vi "PhaseNoise.vi"() -> ()   [LabVIEW 2009]
uses:
  <vilib>/imath/engines/lvmath2/RunTimeEngine/ErrorHandling/NIMS_Finalize Error.vi
  <vilib>/imath/engines/lvmath2/RunTimeEngine/Parser/MC_Version.vi
  <vilib>/imath/engines/lvmath2/RunTimeEngine/NodeEndStatement/NIMS_NodeEndStatement_Output.vi
  <instcachedir>/0/NIMS_NodeEndStatement_Output_53EC0D466D134D7ABD903AC30B43404B.lvgen/NIMS_NodeEndStatement_Output_53EC0D466D134D7ABD903AC30B43404B_001.vi
  <instcachedir>/0/NIMS_NodeEndStatement_Output_53EC0D466D134D7ABD903AC30B43404B.lvgen/NIMS_NodeEndStatement_Output_53EC0D466D134D7ABD903AC30B43404B_000.vi
  <vilib>/imath/engines/lvmath/Functions/Error Handling/MergeErrorsWrapper.vi
  <vilib>/imath/engines/lvmath2/RunTimeEngine/NodeEndStatement/NIMS_NodeEndStatement_Get Vector.vi
  <instcachedir>/0/NIMS_NodeEndStatement_Get Vector_708AE642CFEE4B9892E482CBBBA3A4D6.lvgen/NIMS_NodeEndStatement_Get Vector_708AE642CFEE4B9892E482CBBBA3A4D6_001.vi
  <vilib>/imath/engines/lvmath/Plug In/_Char/NIMS_CH_character datatype.ctl
  <vilib>/imathl/engines/lvmath/Functions/Error Handling/Create Error.vi
  <vilib>/imath/engines/lvmath2/RunTimeEngine/BuiltInFunctions/random/NIMS_random.vi
  <vilib>/imath/engines/lvmath/Plug In/_Char/NIMS_CH_Character RV to String.vi
  <vilib>/imath/engines/lvmath2/RunTimeEngine/RangeToken/NIMS_Range.vi
  <instcachedir>/0/NIMS_Range_08574DECC23E450FAF0AC0BC39E6BEA7.lvgen/NIMS_Range_08574DECC23E450FAF0AC0BC39E6BEA7_001.vi
  <vilib>/imath/engines/lvmath/Functions/Error Handling/MC_Error Cluster From Error Code.vi
  <vilib>/imath/engines/lvmath2/RunTimeEngine/BuiltInFunctions/fft/NIMS_fft(GV).vi
  <instcachedir>/0/NIMS_fft(GV)_4C6467FC22F84E4BA42517A07EF978B0.lvgen/NIMS_fft(GV)_4C6467FC22F84E4BA42517A07EF978B0_001.vi
  <vilib>/imath/engines/lvmath2/RunTimeEngine/BuiltInFunctions/abs/NIMS_abs(signed).vi
  <instcachedir>/0/NIMS_abs(signed)_C4FCB8E6058B49B797C7C8D53CA5F6EC.lvgen/NIMS_abs(signed)_C4FCB8E6058B49B797C7C8D53CA5F6EC_000.vi
  <vilib>/imath/engines/lvmath2/RunTimeEngine/VariableToken/Read/NIMS_Get Elements - RV(_) - Check(_).vi
  <instcachedir>/0/NIMS_Get Elements - RV(_) - Check(_)_FD08F12CA9A340B3A4DC1D5FF02404A0.lvgen/NIMS_Get Elements - RV(_) - Check(_)_FD08F12CA9A340B3A4DC1D5FF02404A0_001.vi
  <vilib>/imath/engines/lvmath2/RunTimeEngine/VariableToken/Read/NIMS_Get Elements - RV(_) - Check.vi
  <instcachedir>/0/NIMS_Get Elements - RV(_) - Check_30A5434E2C4242B098C990FE3FB371BC.lvgen/NIMS_Get Elements - RV(_) - Check_30A5434E2C4242B098C990FE3FB371BC_001.vi
  <instcachedir>/0/NIMS_Get Elements - RV(_) - Check(_)_FD08F12CA9A340B3A4DC1D5FF02404A0.lvgen/NIMS_Get Elements - RV(_) - Check(_)_FD08F12CA9A340B3A4DC1D5FF02404A0_002.vi
  <instcachedir>/0/NIMS_Get Elements - RV(_) - Check_30A5434E2C4242B098C990FE3FB371BC.lvgen/NIMS_Get Elements - RV(_) - Check_30A5434E2C4242B098C990FE3FB371BC_002.vi
  <vilib>/imath/engines/lvmath2/RunTimeEngine/ArithmeticOperatorToken/NIMS_ArithmeticOperator_plus.vi
  <instcachedir>/0/NIMS_ArithmeticOperator_plus_48B9519178ED42D7840F01273E784BFE.lvgen/NIMS_ArithmeticOperator_plus_48B9519178ED42D7840F01273E784BFE_008.vi
  <vilib>/imath/engines/lvmath2/RunTimeEngine/BuiltInFunctions/fft/NIMS_fft(GM).vi
  <instcachedir>/0/NIMS_fft(GM)_D61006EB97DF48D4B7BC0A22887DF931.lvgen/NIMS_fft(GM)_D61006EB97DF48D4B7BC0A22887DF931_000.vi
  <instcachedir>/0/NIMS_abs(signed)_C4FCB8E6058B49B797C7C8D53CA5F6EC.lvgen/NIMS_abs(signed)_C4FCB8E6058B49B797C7C8D53CA5F6EC_002.vi
panel:
  out "Total Power (Watt)":dbl
  out "Power Imbalance (dB)":dbl
  out "Total Power (dB)":dbl
  out "Voltage Imbalance (dB)":dbl
  out "Signal + Noise Power (dB)":dbl[](graph)
  out "Signal Power (Watts)":dbl[](graph)
  out "Signal (Time Domain)":dbl[](graph)
  in  "N1":dbl=64.0
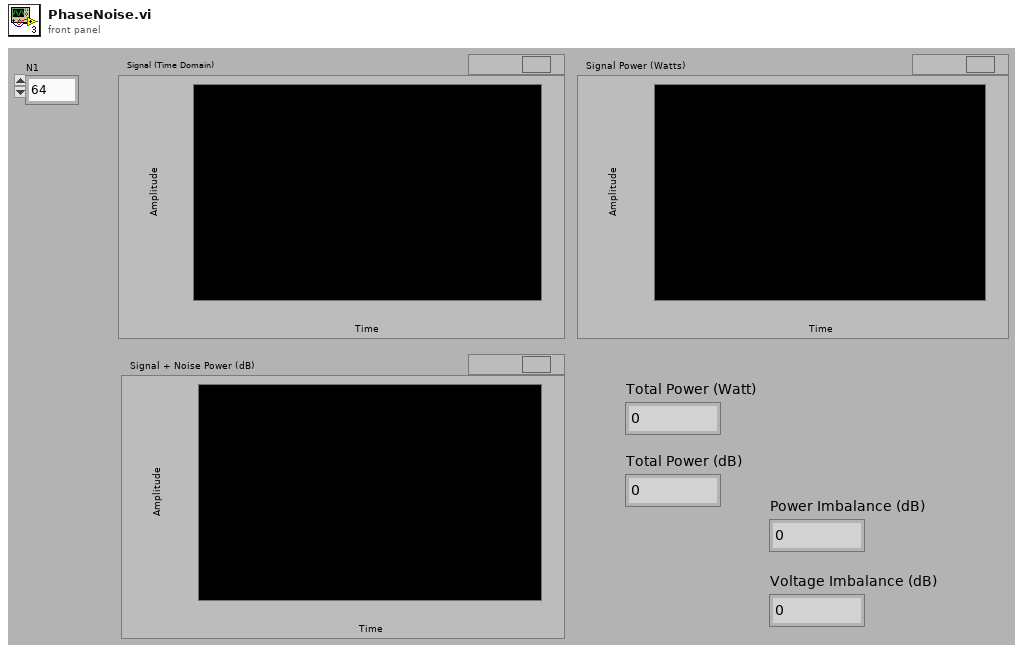
[diagram p1: front panel]
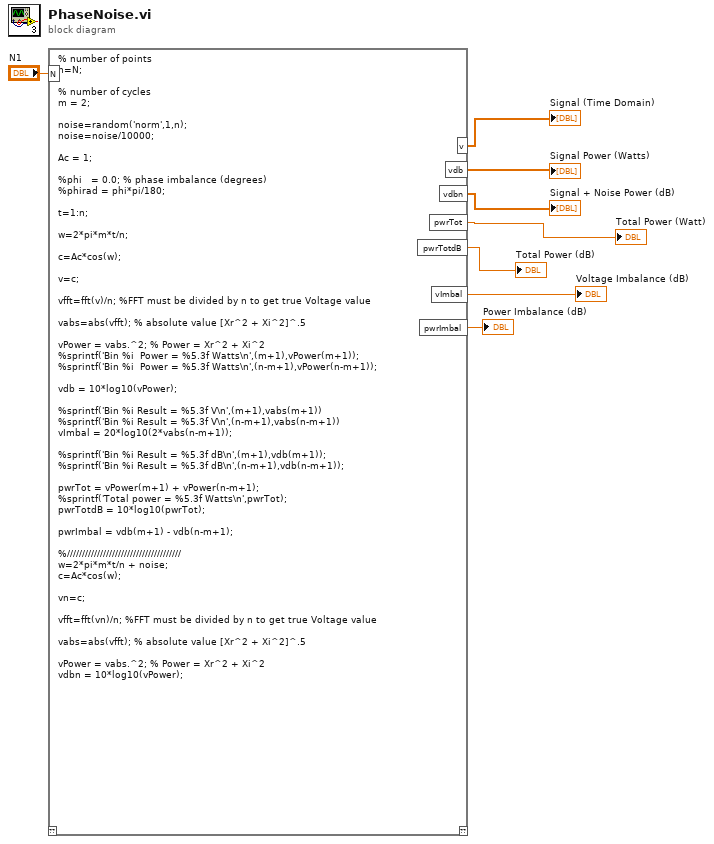
[diagram p0: block diagram]
diagram:
  n1 = mathscript code="% number of points\nn=N;\n\n% number of cycles\nm = 2;\n\nnoise=random('norm',1,n);\nnoise=noise/10000;\n\nAc = 1;\n\n%phi   = 0.0; % phase imbalance (degrees)\n%phirad = phi*pi/180;\n\nt=1:n;\n\nw=2*pi*m*t/n;\n\nc=Ac*cos(w);\n\nv=c;\n\nvfft=fft(v)/n; %FFT must be divided by n to get true Voltage value\n\nvabs=abs(vfft); % absolute value [Xr^2 + Xi^2]^.5\n\nvPower = vabs.^2; % Power = Xr^2 + Xi^2\n%sprintf('Bin %i  Power = %5.3f Watts\\n',(m+1),vPower(m+1));\n%sprintf('Bin %i  Power = %5.3f Watts\\n',(n-m+1),vPower(n-m+1));\n\nvdb = 10*log10(vPower);\n\n%sprintf('Bin %i Result = %5.3f V\\n',(m+1),vabs(m+1))\n%sprintf('Bin %i Result = %5.3f V\\n',(n-m+1),vabs(n-m+1))\nvImbal = 20*log10(2*vabs(n-m+1));\n\n%sprintf('Bin %i Result = %5.3f dB\\n',(m+1),vdb(m+1));\n%sprintf('Bin %i Result = %5.3f dB\\n',(n-m+1),vdb(n-m+1));\n\npwrTot = vPower(m+1) + vPower(n-m+1);\n%sprintf('Total power = %5.3f Watts\\n',pwrTot);\npwrTotdB = 10*log10(pwrTot);\n\npwrImbal = vdb(m+1) - vdb(n-m+1);\n\n%//////////////////////////////////////\nw=2*pi*m*t/n + noise;\nc=Ac*cos(w);\n\nvn=c;\n\nvfft=fft(vn)/n; %FFT must be divided by n to get true Voltage value\n\nvabs=abs(vfft); % absolute value [Xr^2 + Xi^2]^.5\n\nvPower = vabs.^2; % Power = Xr^2 + Xi^2\nvdbn = 10*log10(vPower);"("N"="N1") -> ("v"=→"Signal (Time Domain)":dbl[], "vdbn"=→"Signal + Noise Power (dB)":dbl[], "vdb"=→"Signal Power (Watts)":dbl[], "pwrTotdB"=→"Total Power (dB)":dbl, "vImbal"=→"Voltage Imbalance (dB)":dbl, "pwrImbal"=→"Power Imbalance (dB)":dbl, "pwrTot"=→"Total Power (Watt)":dbl)  [unwired: 1 in, 1 out]
